vi "CameraSobelEdgeDetection.vi"() -> (4 "图像时间戳":u32=16532020 format="%_32g")   [LabVIEW 2015]
uses:
  <vilib>/Analysis/baseanly.llb/Mean (DBL).vi
  <vilib>/Instr/_visa.llb/VISA Configure Serial Port (Instr).vi
  MVCAMSDK.dll
  <vilib>/Analysis/NI_AALBase.lvlib
  <vilib>/vision/NI_Vision_Development_Module.lvlib
panel:
  out "实时循环时间":u32=16532020 format="%_32g"
  in  "平移前进 2":T1=TRUE
  in  "平移计数 2":u16
  in  "平移一次脉冲数 2":u16=20
  out "连接的字符串 2":string
  out "平移信号曲线 2":cluster{"Locations":dbl[], "Amplitudes":dbl[]}[](graph)
  out "连接的字符串":string
  out "转动信号曲线":cluster{"Locations":dbl[], "Amplitudes":dbl[]}[](graph)
  in  "平移回退":T1=TRUE
  in  "转动回退":T1=TRUE
  in  "转动计数":u16
  in  "转动一次脉冲数":u16=20
  in  "转动前进":T1=TRUE
  in  "平移一次脉冲数":u16=20
  in  "平移计数":u16
  in  "flow control (0:none)":u16(ring) caption="流控制（0:无）" items=["无", "XON/XOFF", "RTS/CTS", "XON/XOFF & RTS/CTS", "DTR/DSR", "XON/XOFF & DTR/DSR"]
  in  "stop bits (10: 1 bit)":u16=10 caption="停止位（10: 1位）"
  in  "奇偶 (0:none)":enum16{"None", "Odd", "Even", "Mark", "Space"}(ring) caption="奇偶（0:无）"
  in  "数据比特(默认8)":u16(ring)=8 items=["5"=5, "6"=6, "7"=7, "8"=8]
  in  "波特率(默认9600)":u32=9600
  in  "端口":refnum<visa-resource-name>="COM1"
  in  "平移前进":T1=TRUE
  out "泰伯距离数值":dbl[](array[numeric])=[15.393849374426454, 15.239052716055017, 15.197063981826837, 15.002070246239633]
  out "Locations":dbl[](array[numeric])=[10.438621227921368, 25.832470602347822, 41.07152331840284, 56.268587300229676, 71.27065754646931] caption="上面图像曲线波峰位置"
  out "平移信号曲线":cluster{"Locations":dbl[], "Amplitudes":dbl[]}[](graph)
  out "相机图像":T2(plugin-control)
  out "帧速":u32
  out "帧间耗时\n单位：（0.1ms）":u32
  in  "相机枚举":T3(ring)
  in  "自动曝光模式":bool=TRUE caption="软触发"
  in  "手动曝光模式":bool caption="软触发"
  in  "曝光时间，单位微秒":dbl=11000.0 format="%#_6f"
  in  "硬触发模式":bool caption="软触发"
  in  "软触发模式":bool caption="软触发"
  in  "连续模式":bool caption="软触发"
  in  "软触发一帧":bool caption="软触发"
  in  "读取自定义数据":bool
  out "从相机中读出的字符串(32字节)":string
  in  "写入自定义数据":bool
  in  "要写入相机的字符串(32字节)":string
  in  "拍照":bool
  in  "相机参数":bool=TRUE
  in  "Stop":bool
  in  "激活预览":bool=TRUE
  out "Image":T2(plugin-control)
  # "相机原生分辨率设置"
  # "写入自定义数据"
  # "触发设置"
  # "曝光设置"
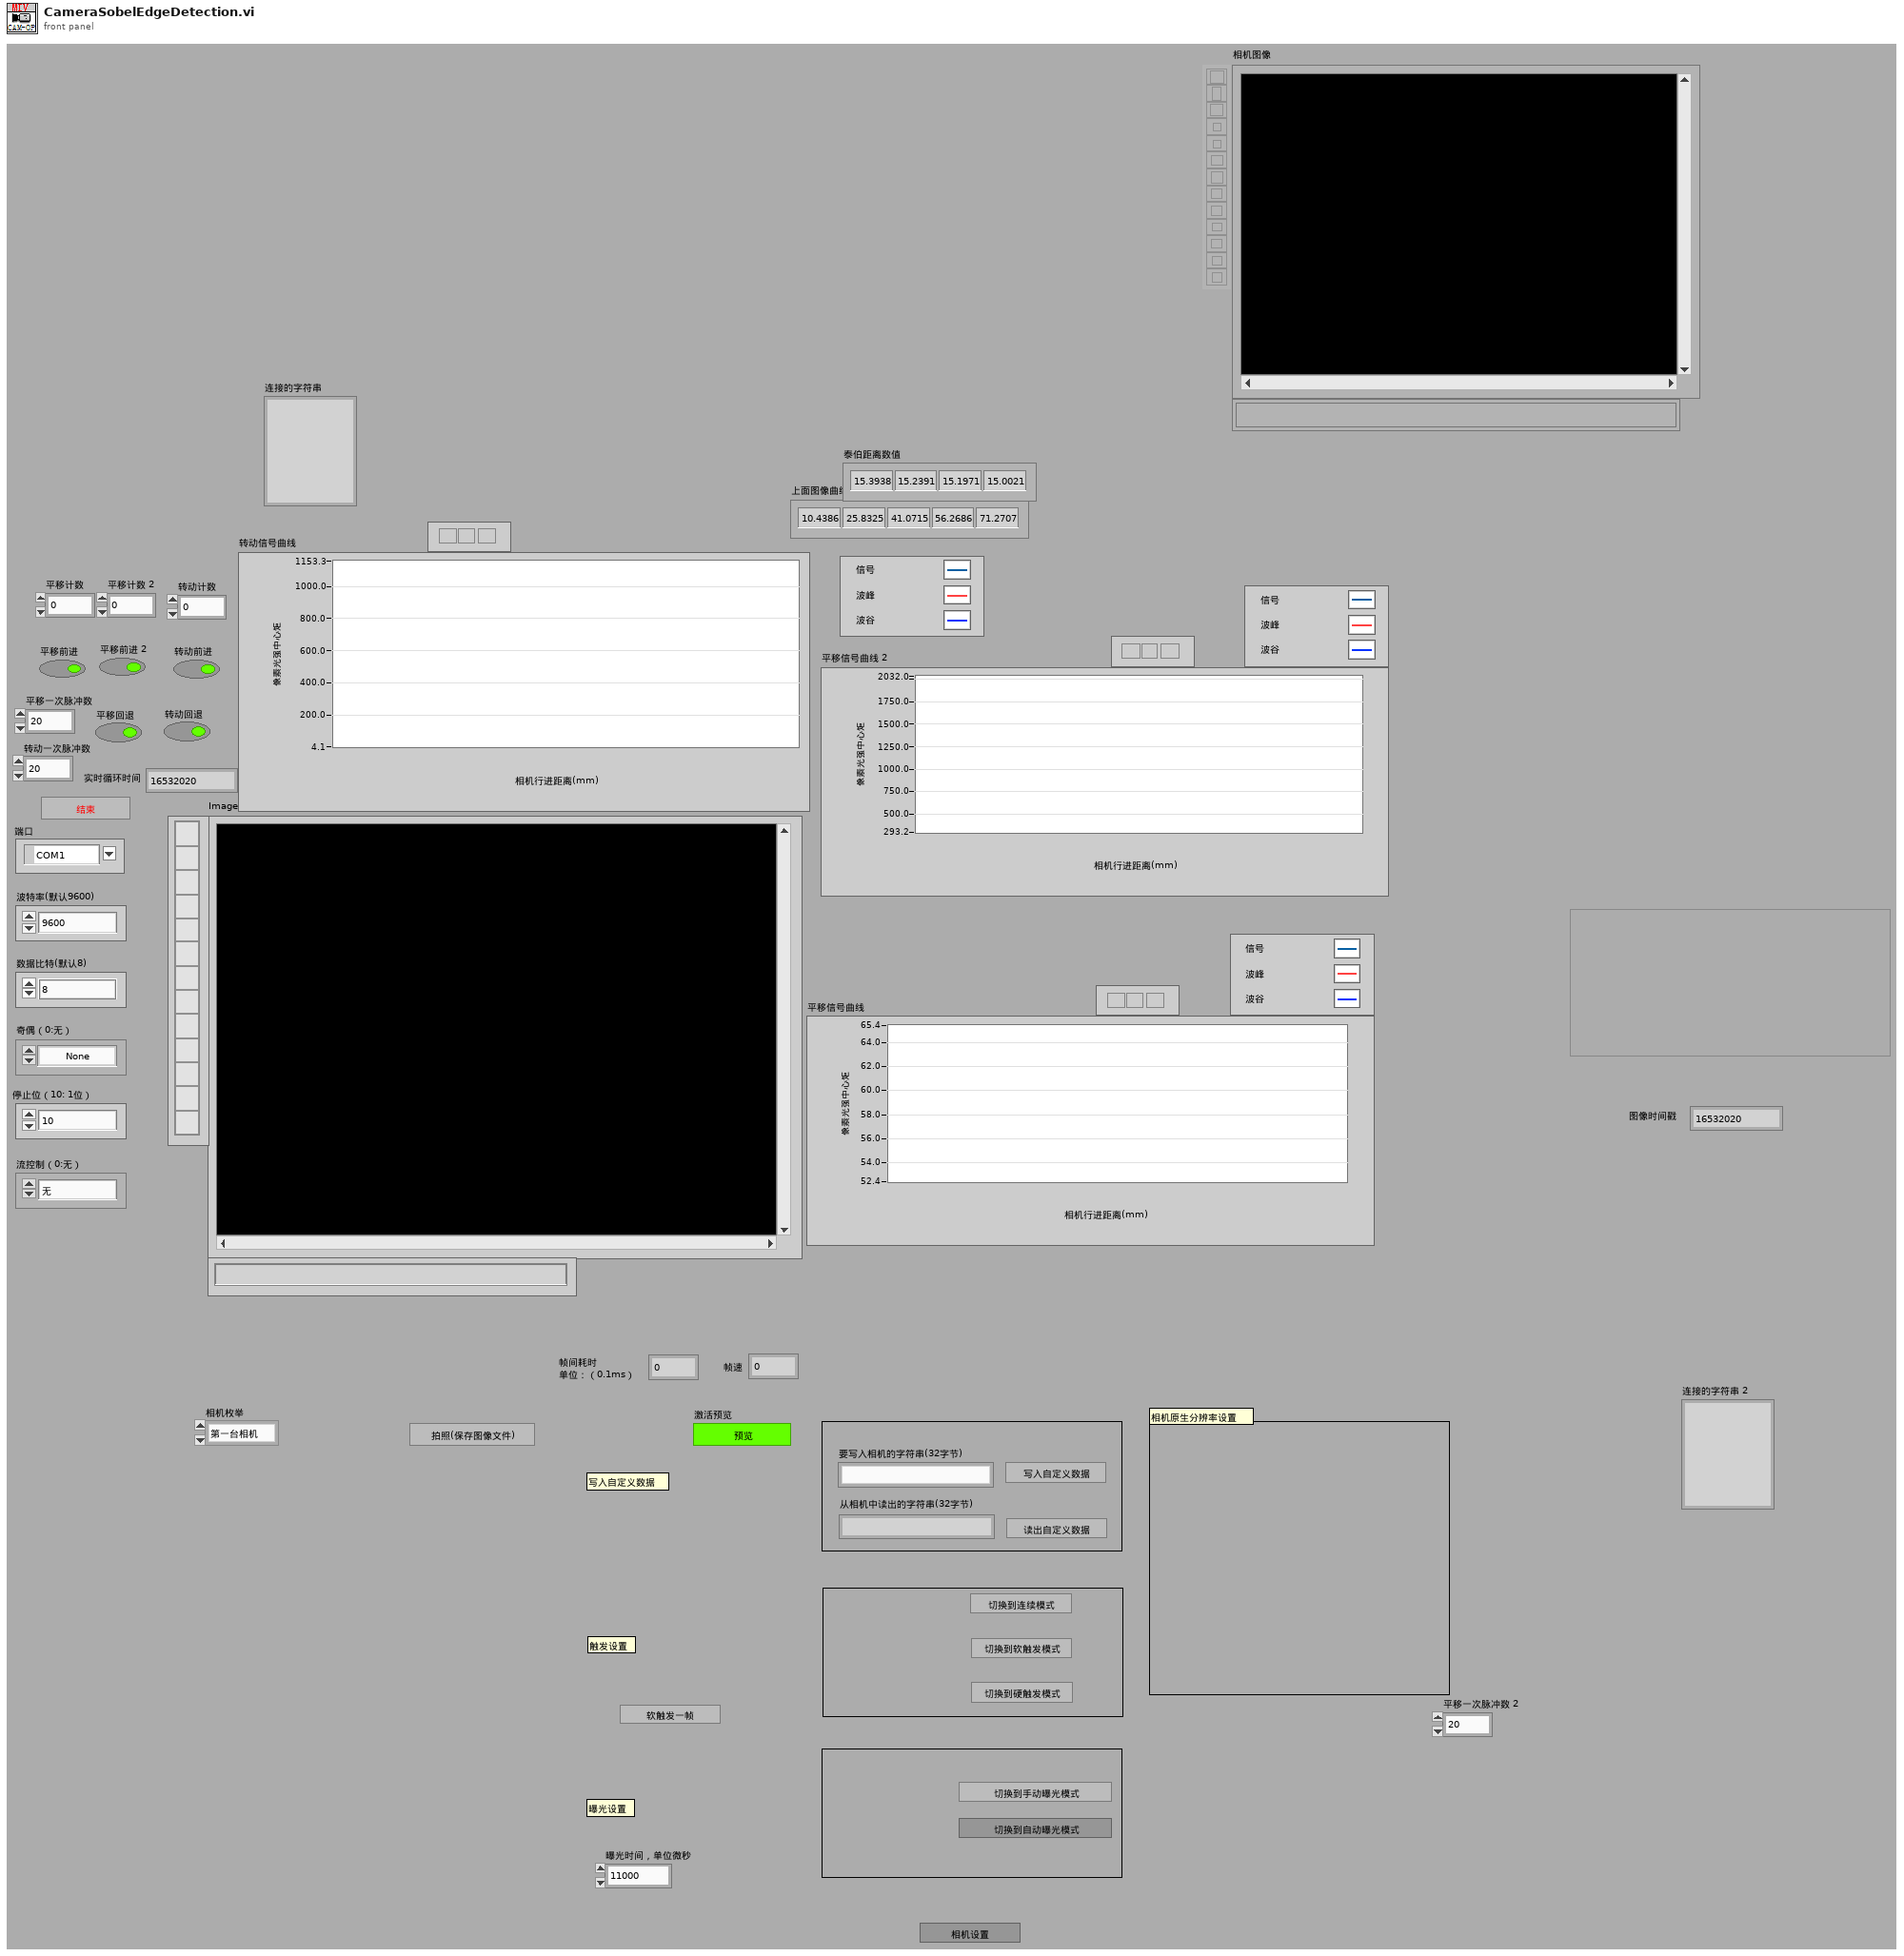
[diagram p1: front panel]
types:
  T1 = typedef "控件 1.ctl" = bool
  T2 = typedef "IMAQ Image.ctl" = refnum<image>
  T3 = enum16{"第一台相机", "第二台相机", "第三台相机", "第四台相机", "第五台相机"}
  T4 = typedef "Image Type" = u32
  T5 = enum32{"Differentiation", "Gradient", "Prewitt", "Roberts", "Sigma", "Sobel"}
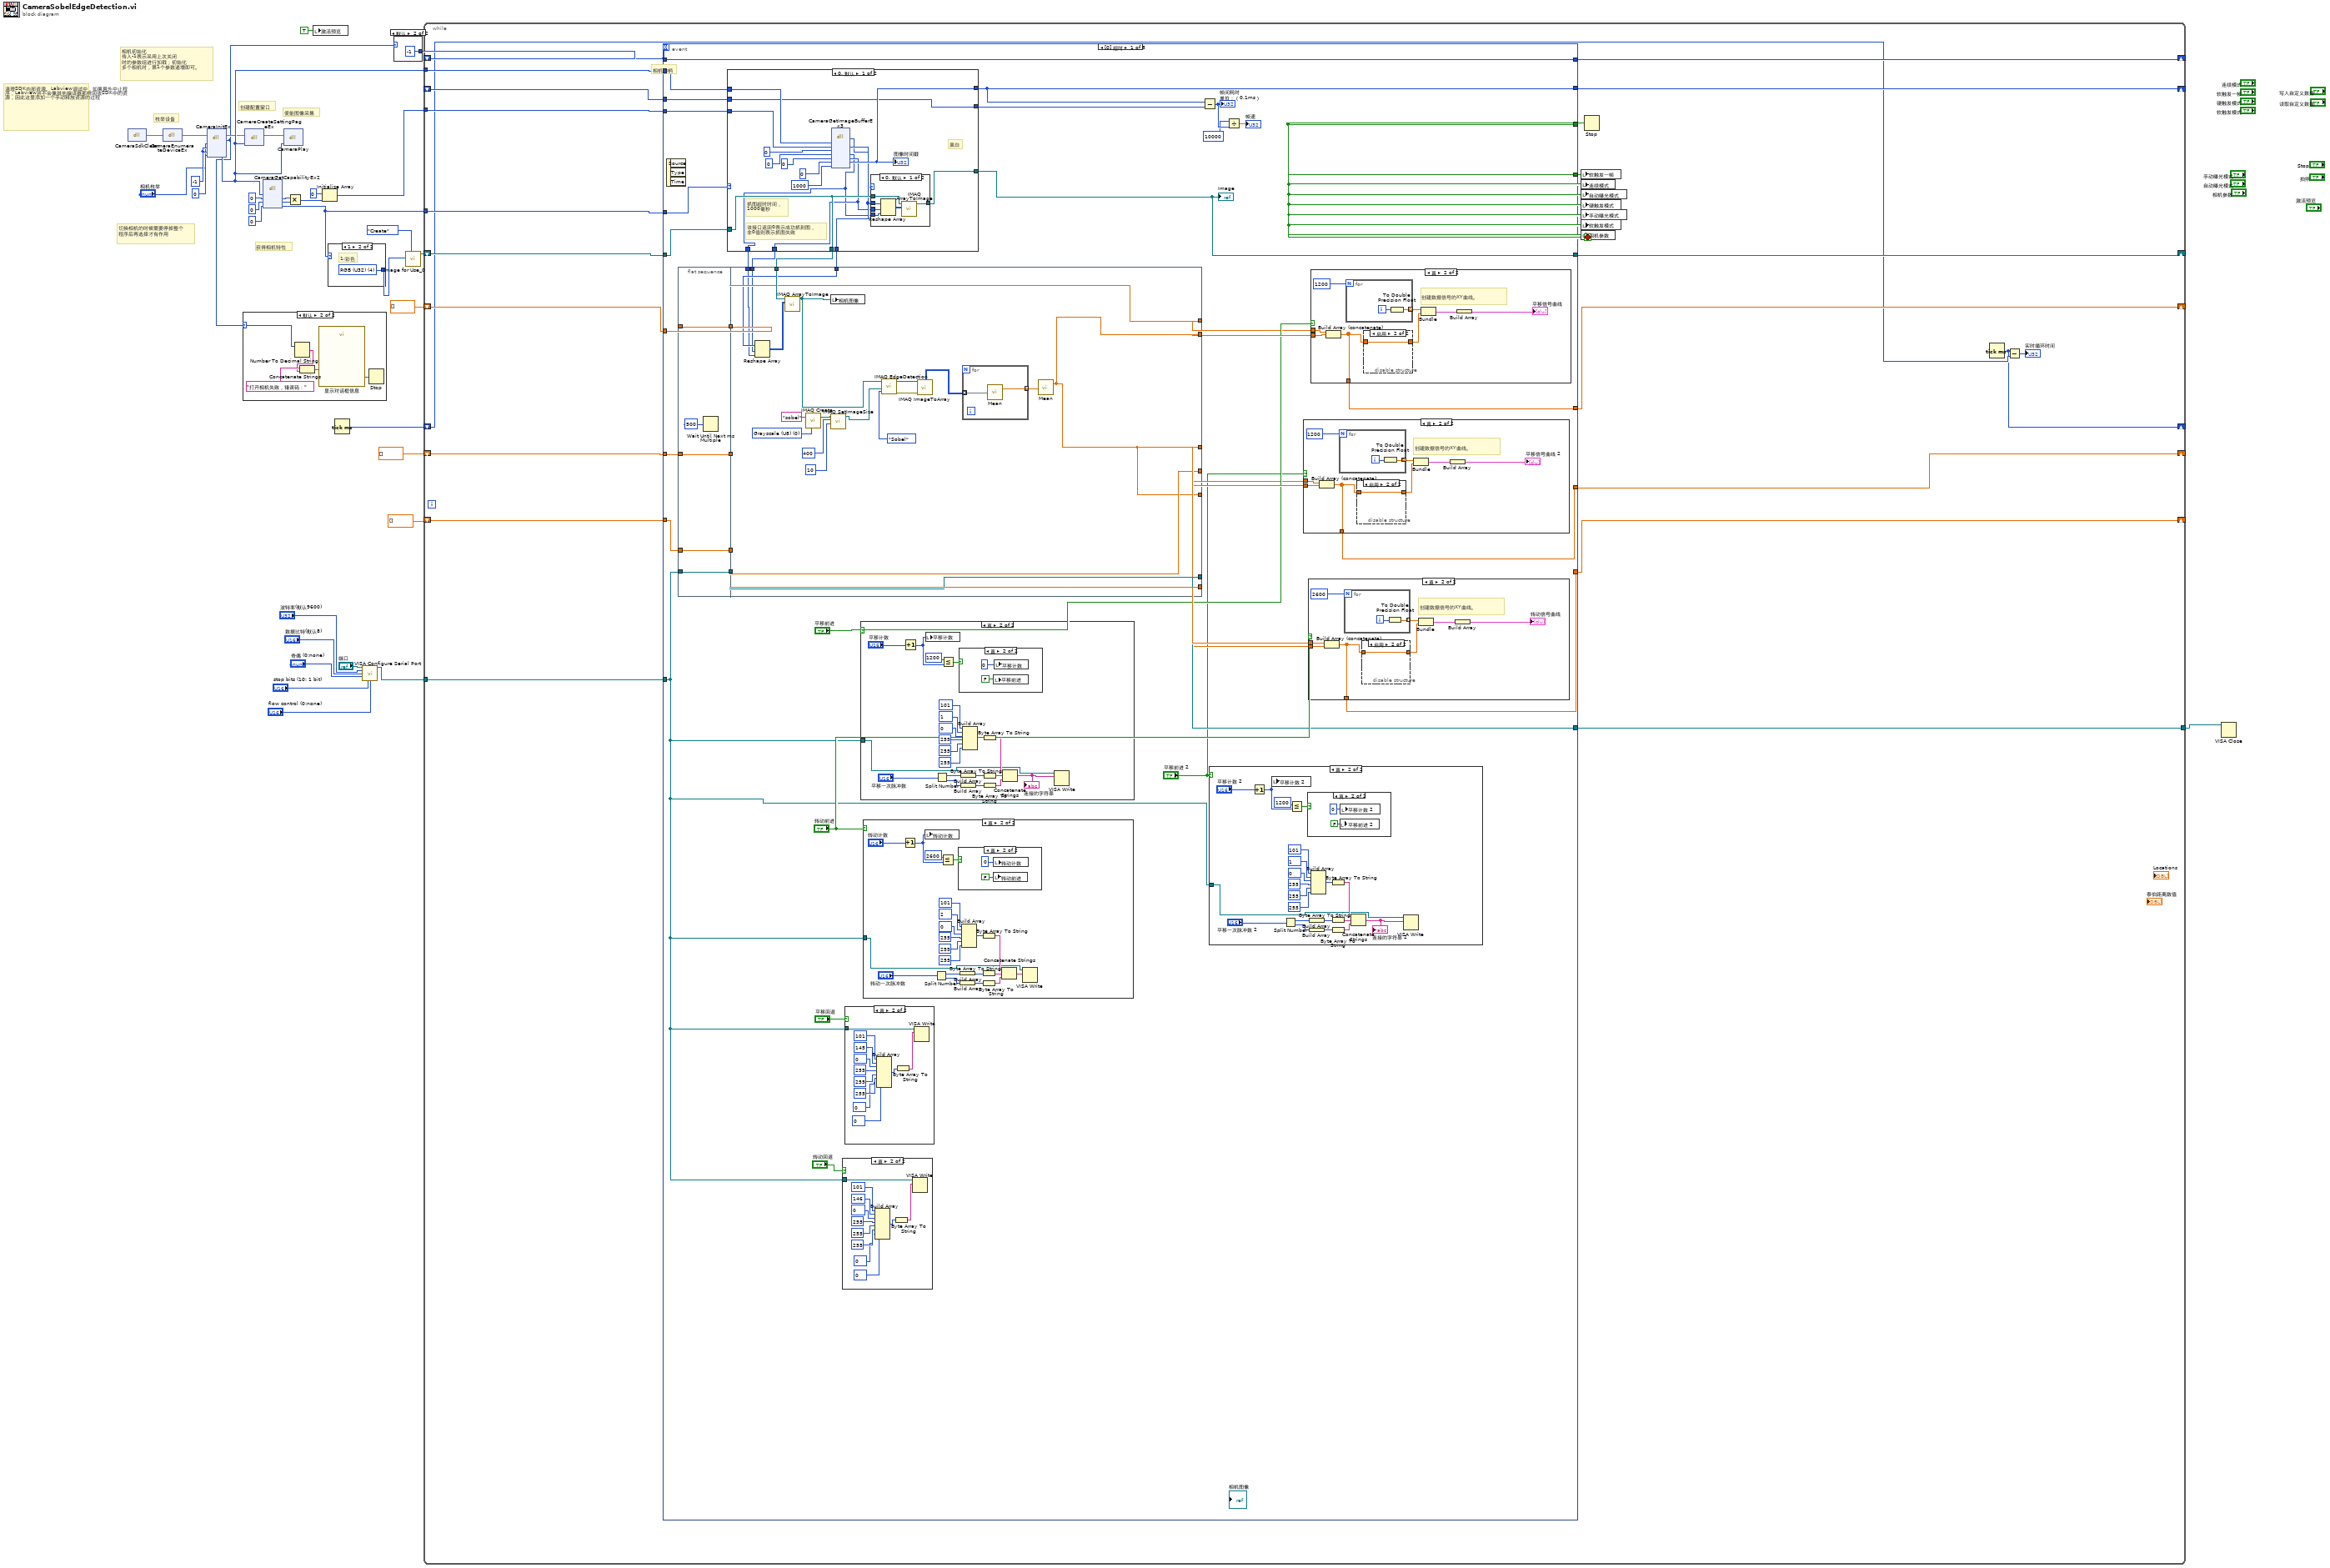
[diagram p0: block diagram]
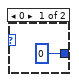
[diagram p2: hidden frame]
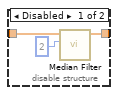
[diagram p7: hidden frame]
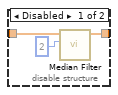
[diagram p9: hidden frame]
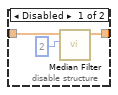
[diagram p11: hidden frame]
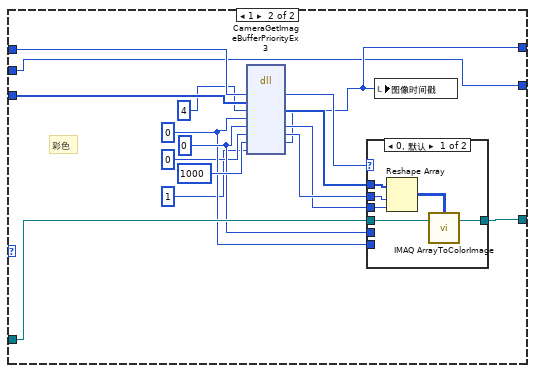
[diagram p19: hidden frame]
diagram:
  w32 = -1
  # "切换相机的时候需要停掉整个\n程序后再选择才有作用"
  # "清理SDK内部资源。Labview调试中，如果意外中止程序，Labview并不会像其他编译器那样回收SDK中的资源，因此这里添加一个手动释放资源的过程"
  # "使能图像采集"
  # "获得相机特性"
  # "创建配置窗口"
  # "相机初始化\n传入-1表示采用上次关闭\n时的参数组进行加载；初始化\n多个相机时，第1个参数递增即可。"
  # "枚举设备"
  n1 = dll-call lib="MVCAMSDK.dll" fn="CameraSdkClean"() -> (error out=w33:errorcluster)  [unwired: 4 in, 1 out]
  n2 = dll-call lib="MVCAMSDK.dll" fn="CameraEnumerateDeviceEx"(error in=w33) -> (error out=w30:errorcluster)  [unwired: 3 in, 1 out]
  n3 = dll-call lib="MVCAMSDK.dll" fn="CameraInitEx"(error in=w30, "相机索引值"="相机枚举", "参数加载方式"=w32, "要加载的参数组索引"=w32, "相机句柄"=0) -> (error out=w19:errorcluster, "返回类型"=w14:i32, "相机句柄"=w21:i32)  [unwired: 5 in, 1 out]
  n4 = case shown="默认" w14 {
    selector: w14 -> [_ w39]
    frame 0 {
    }
    frame Default {
      n5 = Number To Decimal String(number=w39) -> (decimal integer string=w36:string)  [unwired: 1 in]
      n6 = Concatenate Strings("打开相机失败，错误码：" ("字符串"), w36) -> (w38:string)
      n7 = call "显示对话框信息"("Message"=w38) -> ("结束"=w40:bool)  [unwired: 9 in, 1 out]
      n8 = Stop(stop? (T)=w40) -> ()
    }
  }
  n9 = dll-call lib="MVCAMSDK.dll" fn="CameraCreateSettingPageEx"(error in=w19, "相机句柄"=w21) -> (error out=w22:errorcluster)  [unwired: 4 in, 1 out]
  n10 = dll-call lib="MVCAMSDK.dll" fn="CameraGetCapabilityEx2"("相机句柄"=w21, "图像最大宽度"=0, "图像最大高度"=0, "是否是彩色相机(返回0:黑白;1:彩色)"=0) -> ("图像最大宽度"=w24:i32, "图像最大高度"=w23:i32, "是否是彩色相机(返回0:黑白;1:彩色)"=w18:i32)  [unwired: 5 in, 2 out]
  n11 = dll-call lib="MVCAMSDK.dll" fn="CameraPlay"(error in=w22, "相机句柄"=w21) -> ()  [unwired: 4 in, 2 out]
  n12 = Multiply(x=w24, y=w23) -> (x*y=w28:i32)
  n13 = local write "激活预览"(TRUE ("激活预览")) -> ()
  n14 = Initialize Array(0, w28) -> (w20:i32[])
  n15 = case shown="1" w18 {
    tunnel: [_ w41] -> w34
    frame 0, Default {
      # "0:黑白;"
    }
    frame 1 {
      w41 = T4 4 items=["Grayscale (U8)", "Grayscale (I16)", "Grayscale (SGL)", "Complex (CSG)", "RGB (U32)", "HSL (U32)", "RGB (U64)", "Grayscale (U16)"] ("Image Type")
      # "1:彩色"
    }
  }
  n16 = Tick Count (ms)() -> (millisecond timer value=w1:u32)
  n17 = call-poly "VISA Configure Serial Port"("VISA resource name"="端口", "baud rate (9600)"="波特率(默认9600)", "data bits (8)"="数据比特(默认8)", "parity (0:none)"="奇偶 (0:none)", "stop bits (10: 1 bit)"="stop bits (10: 1 bit)", "flow control (0:none)"="flow control (0:none)") -> ("VISA resource name out"=w6:refnum<visa-resource-name>)  [unwired: 8 in, 1 out]
  n18 = case shown="默认" w14 {
    tunnel: [0 -1] -> w13
    frame 0 {
    }
    frame Default {
    }
  }
  n19 = call "Image for Use_0.vi"("Command"=enum16{"Create", "Use", "Copy in", "Dispose"}."Create", "Image Type"=w34) -> ("Image out"=w17:T2)  [unwired: 8 in, 1 out]
  n20 = while {
    tunnel: w21 -> [w62]
    tunnel: w20 -> [w64]
    tunnel: w18 -> [w65]
    shift-right: [w61] -> _
    shift-left: w13 -> [w60]
    shift-right: [w58] -> _
    shift-left: w17 -> [w63]
    shift-right: [w57] -> _
    shift-left: _ -> [w56]
    tunnel: w6 -> [w54]
    tunnel: [w53] -> w5
    shift-right: [w51] -> _
    shift-left: dbl[] [] -> [w52]
    shift-right: [w50] -> _
    shift-left: dbl[] [] -> [w49]
    shift-right: [w47] -> _
    shift-left: dbl[] [] -> [w48]
    shift-right: [w44] -> _
    shift-left: w1 -> [w45]
    stop <- w55 stop-if-true
    # "相机句柄"
    n21 = event shown="[0] 超时" {
      selector: _ -> [_ _ _ _ _ _ _ _]
      dyn-events: _ -> [_ _ _ _ _ _ _ _]
      timeout: w60 -> [_ _ _ _ _ _ _ _]
      tunnel: [_ _ _ _ _ _ _ TRUE] -> w55
      tunnel: w64 -> [w103 _ _ _ _ _ _ _]
      tunnel: w65 -> [w102 _ _ _ _ _ _ _]
      tunnel: w62 -> [w104 _ w323 w341 w356 _ w370 w390]
      tunnel: w63 -> [w101 w316 w322 w340 w355 w360 w369 w388]
      tunnel: [w100 w317 w324 w342 w357 w361 w371 w391] -> w61
      tunnel: w60 -> [w100 _ w324 w342 w357 w361 w371 w391]
      tunnel: [_ _ _ _ _ _ _ FALSE] -> w59
      tunnel: [w99 w316 w322 w340 w355 w360 w369 w388] -> w58
      tunnel: [w96 w315 w321 w339 w354 w359 w368 w387] -> w57
      tunnel: w56 -> [w98 w315 w321 w339 w354 w359 w368 w387]
      tunnel: w54 -> [w69 _ _ _ _ _ _ _]
      tunnel: [w80 _ _ _ _ _ _ _] -> w53
      tunnel: w52 -> [w86 _ _ _ _ _ _ _]
      tunnel: [w89 _ _ _ _ _ _ _] -> w51
      tunnel: [w88 _ _ _ _ _ _ _] -> w50
      tunnel: w49 -> [w82 _ _ _ _ _ _ _]
      tunnel: [w77 _ _ _ _ _ _ _] -> w47
      tunnel: w48 -> [w74 _ _ _ _ _ _ _]
      event Timeout {
        n22 = event-data() -> ()  [unwired: 1 in, 3 out]
        n23 = flat-sequence {
          tunnel: w86 -> [w147]
          tunnel: [w147] -> w85
          tunnel: [w145] -> w83
          tunnel: w82 -> [w145]
          tunnel: [w144] -> w81
          tunnel: w69 -> [w144]
          tunnel: w74 -> [w143]
          tunnel: [w143] -> w73
          tunnel: w92 -> [w169]
          tunnel: [w157] -> w78
          tunnel: [w168] -> w71
          tunnel: w85 -> [w168]
          tunnel: [w167] -> w84
          tunnel: w83 -> [w167]
          tunnel: [w166] -> w80
          tunnel: w81 -> [w166]
          tunnel: [w157] -> w79
          tunnel: [w157] -> w76
          tunnel: w73 -> [w165]
          tunnel: [w165] -> w72
          tunnel: w68 -> [w150]
          tunnel: w67 -> [w149]
          tunnel: w66 -> [w148]
          frame #0 {
            n24 = Wait Until Next ms Multiple(millisecond multiple=u32 500 ("毫秒倍数")) -> ()  [unwired: 1 out]
          }
          frame #1 {
            w156 = T4 0 items=["Grayscale (U8)", "Grayscale (I16)", "Grayscale (SGL)", "Complex (CSG)", "RGB (U32)", "HSL (U32)", "RGB (U64)", "Grayscale (U16)"] ("Image Type")
            n25 = Reshape Array(w150, w149, w148) -> (w151:u8[][])
            n26 = call "IMAQ ArrayToImage"("Image Pixels (U8)"=w151, "Image"=w169) -> ("Image Out"=w160:T2)  [unwired: 8 in, 1 out]
            n27 = call "IMAQ Create"("Image Name"="sobel", "Image Type"=w156) -> ("New Image"=w155:T2)  [unwired: 3 in, 1 out]
            n28 = local write "相机图像"(w160) -> ()
            n29 = call "IMAQ SetImageSize"("Y Resolution"=10, "X Resolution"=400, "Image"=w155) -> ("Image Out"=w154:T2)  [unwired: 2 in, 1 out]
            n30 = call "IMAQ EdgeDetection"("Method"=T5."Sobel", "Image Dst"=w154, "Image Src"=w160) -> ("error out"=w161:errorcluster, "Image Dst Out"=w162:T2)  [unwired: 7 in]
            n31 = call "IMAQ ImageToArray"("error in (no error)"=w161, "Image"=w162) -> ("Image Pixels (U8)"=w159:u8[][])  [unwired: 2 in, 4 out]
            n32 = for {
              tunnel: w159 -> [w171] mode=indexing
              tunnel: [w170] -> w158 mode=indexing
              n33 = call-poly <vilib>:"Mean.vi"("X"=w171) -> ("mean"=w170:dbl)  [unwired: 1 out]
            }
            n34 = call-poly <vilib>:"Mean.vi"("X"=w158) -> ("mean"=w157:dbl)  [unwired: 1 out]
          }
        }
        n35 = case shown="0, 默认" w102 {
          tunnel: w103 -> [w284 w307]
          tunnel: w101 -> [w274 w306]
          tunnel: w104 -> [w277 w305]
          tunnel: [w278 w295] -> w99
          tunnel: [w276 w294] -> w96
          tunnel: w98 -> [w275 w293]
          tunnel: [w275 w293] -> w97
          tunnel: [w274 _] -> w92
          tunnel: [w273 _] -> w68
          tunnel: [w271 _] -> w67
          tunnel: [w270 _] -> w66
          frame 0, Default {
            # "黑白"
            # "该接口返回0表示成功抓到图，\n非0值则表示抓图失败"
            # "抓图超时时间，\n1000毫秒"
            n36 = dll-call lib="MVCAMSDK.dll" fn="CameraGetImageBufferEx3"("相机句柄"=w277, "图像数据缓冲区"=w284, "图像输出格式(0:8位灰度;1:24位彩色;2:32位彩色，3：BGR24彩色 4：BGRA32位彩色)"=0, "图像宽度"=0, "图像高度"=0, "时间戳(单位为100微秒)"=0, "抓图超时时间(毫秒)"=1000) -> ("返回类型"=w272:i32, "图像数据缓冲区"=w273:u8[], "图像宽度"=w270:i32, "图像高度"=w271:i32, "时间戳(单位为100微秒)"=w276:u32)  [unwired: 6 in, 2 out]
            "图像时间戳" <- w276
            n37 = case shown="0, 默认" w272 {
              tunnel: w273 -> [w290 _]
              tunnel: w274 -> [w287 w291]
              tunnel: w271 -> [w289 _]
              tunnel: w270 -> [w288 _]
              tunnel: [w285 w291] -> w278
              frame 0, Default {
                n38 = Reshape Array(w290, w289, w288) -> (w286:u8[][])
                n39 = call "IMAQ ArrayToImage"("Image Pixels (U8)"=w286, "Image"=w287) -> ("Image Out"=w285:T2)  [unwired: 8 in, 1 out]
              }
              frame -12 {
              }
            }
          }
          frame 1 {
            w297 = 0
            w298 = 0
            # "彩色"
            n40 = dll-call lib="MVCAMSDK.dll" fn="CameraGetImageBufferPriorityEx3"("相机句柄"=w305, "图像数据缓冲区"=w307, "图像输出格式(0:8位灰度;1:24位彩色;2:32位彩色)"=4, "图像宽度"=w297, "图像高度"=w298, "时间戳（单位为100微秒）"=0, "抓图超时时间(毫秒)"=1000, "取图优先级(0: 取最旧   1:取最新)"=1) -> ("返回类型"=w299:i32, "图像数据缓冲区"=w302:u32[], "图像宽度"=w300:i32, "图像高度"=w301:i32, "时间戳（单位为100微秒）"=w294:u32)  [unwired: 7 in, 2 out]
            n41 = case shown="0, 默认" w299 {
              tunnel: w302 -> [w312 _]
              tunnel: w306 -> [w311 w314]
              tunnel: w301 -> [w310 _]
              tunnel: w300 -> [w309 _]
              tunnel: w298 -> [_ _]
              tunnel: w297 -> [_ _]
              tunnel: [w308 w314] -> w295
              frame 0, Default {
                n42 = Reshape Array(w312, w310, w309) -> (w313:u32[][])
                n43 = call "IMAQ ArrayToColorImage"("Image Pixels (U32)"=w313, "Image"=w311) -> ("Image Out"=w308:T2)  [unwired: 3 in, 1 out]
              }
              frame -12 {
              }
            }
            n44 = local write "图像时间戳"(w294) -> ()
          }
        }
        "Image" <- w99
        n45 = case shown="真" "转动回退" {
          tunnel: w69 -> [_ w205]
          frame False {
          }
          frame True {
            n46 = Build Array(101, 146, 0, 255, 255, 255, 0, 0) -> (w206:i32[])
            n47 = Byte Array To String(unsigned byte array=w206) -> (string=w204:string)
            n48 = VISA Write(VISA resource name=w205, write buffer=w204) -> ()  [unwired: 1 in, 3 out]
          }
        }
        n49 = case shown="真" "平移回退" {
          tunnel: w69 -> [_ w216]
          frame False {
          }
          frame True {
            n50 = Build Array(101, 145, 0, 255, 255, 255, 0, 0) -> (w217:i32[])
            n51 = Byte Array To String(unsigned byte array=w217) -> (string=w215:string)
            n52 = VISA Write(VISA resource name=w216, write buffer=w215) -> ()  [unwired: 1 in, 3 out]
          }
        }
        n53 = case shown="真" "平移前进" {
          tunnel: w69 -> [_ w250]
          frame False {
          }
          frame True {
            n54 = Increment(x="平移计数") -> (x+1=w248:u16)
            n55 = local write "平移计数"(w248) -> ()
            n56 = Split Number(x="平移一次脉冲数") -> (hi(x)=w258:u8, lo(x)=w257:u8)
            n57 = Less Or Equal?(x=1200, y=w248) -> (x <= y?=w260:bool)
            n58 = case shown="真" w260 {
              frame False {
              }
              frame True {
                n59 = local write "平移前进"(T1 FALSE ("平移前进")) -> ()
                n60 = local write "平移计数"(u16 0 ("平移计数 2")) -> ()
              }
            }
            n61 = Build Array(w258) -> (w256:u8[])
            n62 = Build Array(w257) -> (w255:u8[])
            n63 = Build Array(101, 1, 0, 255, 255, 255) -> (w254:i32[])
            n64 = Byte Array To String(unsigned byte array=w254) -> (string=w253:string)
            n65 = Byte Array To String(unsigned byte array=w256) -> (string=w252:string)
            n66 = Byte Array To String(unsigned byte array=w255) -> (string=w251:string)
            n67 = Concatenate Strings(w253, w252, w251) -> (w247:string)
            "连接的字符串" <- w247
            n68 = VISA Write(VISA resource name=w250, write buffer=w247) -> ()  [unwired: 1 in, 3 out]
          }
        }
        n69 = case shown="真" "转动前进" {
          tunnel: w69 -> [_ w228]
          frame False {
          }
          frame True {
            n70 = Increment(x="转动计数") -> (x+1=w226:u16)
            n71 = local write "转动计数"(w226) -> ()
            n72 = Split Number(x="转动一次脉冲数") -> (hi(x)=w236:u8, lo(x)=w235:u8)
            n73 = Less Or Equal?(x=2600, y=w226) -> (x <= y?=w238:bool)
            n74 = case shown="真" w238 {
              frame False {
              }
              frame True {
                n75 = local write "转动前进"(T1 FALSE ("平移前进")) -> ()
                n76 = local write "转动计数"(u16 0 ("平移计数")) -> ()
              }
            }
            n77 = Build Array(w236) -> (w234:u8[])
            n78 = Build Array(w235) -> (w233:u8[])
            n79 = Build Array(101, 2, 0, 255, 255, 255) -> (w232:i32[])
            n80 = Byte Array To String(unsigned byte array=w232) -> (string=w231:string)
            n81 = Byte Array To String(unsigned byte array=w234) -> (string=w230:string)
            n82 = Byte Array To String(unsigned byte array=w233) -> (string=w229:string)
            n83 = Concatenate Strings(w231, w230, w229) -> (w225:string)
            n84 = VISA Write(VISA resource name=w228, write buffer=w225) -> ()  [unwired: 1 in, 3 out]
          }
        }
        n85 = Subtract(x=w96, y=w97) -> (x-y=w95:u32)
        "帧间耗时\n单位：（0.1ms）" <- w95
        n86 = case shown="真" "平移前进 2" {
          tunnel: w69 -> [_ w108]
          frame False {
          }
          frame True {
            n87 = Increment(x="平移计数 2") -> (x+1=w106:u16)
            n88 = local write "平移计数 2"(w106) -> ()
            n89 = Split Number(x="平移一次脉冲数 2") -> (hi(x)=w116:u8, lo(x)=w115:u8)
            n90 = Less Or Equal?(x=1200, y=w106) -> (x <= y?=w118:bool)
            n91 = case shown="真" w118 {
              frame False {
              }
              frame True {
                n92 = local write "平移前进 2"(T1 FALSE ("平移前进")) -> ()
                n93 = local write "平移计数 2"(u16 0 ("平移计数 2")) -> ()
              }
            }
            n94 = Build Array(w116) -> (w114:u8[])
            n95 = Build Array(w115) -> (w113:u8[])
            n96 = Build Array(101, 1, 0, 255, 255, 255) -> (w112:i32[])
            n97 = Byte Array To String(unsigned byte array=w112) -> (string=w111:string)
            n98 = Byte Array To String(unsigned byte array=w114) -> (string=w110:string)
            n99 = Byte Array To String(unsigned byte array=w113) -> (string=w109:string)
            n100 = Concatenate Strings(w111, w110, w109) -> (w105:string)
            "连接的字符串 2" <- w105
            n101 = VISA Write(VISA resource name=w108, write buffer=w105) -> ()  [unwired: 1 in, 3 out]
          }
        }
        n102 = Divide(x=u32 10000 ("帧间耗时"), y=w95) -> (x/y=→"帧速":dbl)
        n103 = case shown="真" "平移前进 2" {
          tunnel: w72 -> [w128 w131]
          tunnel: w76 -> [_ w129]
          tunnel: [w128 w130] -> w77
          frame False {
          }
          frame True {
            # "创建数据信号的XY曲线。"
            n104 = Build Array (concatenate)(w131, w129) -> (w130:dbl[])
            n105 = for {
              N: i64 1200 ("数值") -> [_]
              tunnel: [w137] -> w135 mode=indexing
              i -> [w138]
              n106 = To Double Precision Float(number=w138) -> (double precision float=w137:dbl)
            }
            n107 = disable-structure shown="启用" {
              disable-tunnel: w130 -> [w140 w142]
              disable-tunnel: [w139 w142] -> w134
              frame Disabled {
                n108 = call <vilib>:"Median Filter.vi"("left rank"=2, "X"=w140) -> ("Filtered X"=w139:dbl[])  [unwired: 8 in, 1 out]
              }
              frame Enabled {
              }
            }
            n109 = Bundle(w135, w134) -> (w132:cluster{dbl[], dbl[]})  [unwired: 1 in]
            n110 = Build Array(w132) -> (→"平移信号曲线 2":cluster{dbl[], dbl[]}[])
          }
        }
        n111 = case shown="真" "转动前进" {
          tunnel: w79 -> [_ w175]
          tunnel: w84 -> [w172 w174]
          tunnel: [w172 w173] -> w88
          frame False {
          }
          frame True {
            # "创建数据信号的XY曲线。"
            n112 = Build Array (concatenate)(w174, w175) -> (w173:dbl[])
            n113 = for {
              N: i64 2600 ("数值") -> [_]
              tunnel: [w181] -> w177 mode=indexing
              i -> [w182]
              n114 = To Double Precision Float(number=w182) -> (double precision float=w181:dbl)
            }
            n115 = disable-structure shown="启用" {
              disable-tunnel: w173 -> [w184 w186]
              disable-tunnel: [w183 w186] -> w178
              frame Disabled {
                n116 = call <vilib>:"Median Filter.vi"("left rank"=2, "X"=w184) -> ("Filtered X"=w183:dbl[])  [unwired: 8 in, 1 out]
              }
              frame Enabled {
              }
            }
            n117 = Bundle(w177, w178) -> (w180:cluster{dbl[], dbl[]})  [unwired: 1 in]
            n118 = Build Array(w180) -> (→"转动信号曲线":cluster{dbl[], dbl[]}[])
          }
        }
        n119 = case shown="真" "平移前进" {
          tunnel: w71 -> [w187 w189]
          tunnel: w78 -> [_ w190]
          tunnel: [w187 w188] -> w89
          frame False {
          }
          frame True {
            # "创建数据信号的XY曲线。"
            n120 = Build Array (concatenate)(w189, w190) -> (w188:dbl[])
            n121 = for {
              N: i64 1200 ("数值") -> [_]
              tunnel: [w196] -> w194 mode=indexing
              i -> [w197]
              n122 = To Double Precision Float(number=w197) -> (double precision float=w196:dbl)
            }
            n123 = disable-structure shown="启用" {
              disable-tunnel: w188 -> [w199 w201]
              disable-tunnel: [w198 w201] -> w193
              frame Disabled {
                n124 = call <vilib>:"Median Filter.vi"("left rank"=2, "X"=w199) -> ("Filtered X"=w198:dbl[])  [unwired: 8 in, 1 out]
              }
              frame Enabled {
              }
            }
            n125 = Bundle(w194, w193) -> (w191:cluster{dbl[], dbl[]})  [unwired: 1 in]
            n126 = Build Array(w191) -> (→"平移信号曲线":cluster{dbl[], dbl[]}[])
          }
        }
      }
      event "激活预览": Value Change {
        n127 = event-data() -> ("NewVal"=w318:bool)  [unwired: 1 in, 5 out]
        n128 = case shown="真" w318 {
          tunnel: [-1 0] -> w317
          frame False {
          }
          frame True {
          }
        }
      }
      event "连续模式", "软触发一帧", "硬触发模式", "软触发模式": Value Change {
        n129 = event-data() -> ("CtlRef"=w326:refnum<vi>)  [unwired: 1 in, 5 out]
        n130 = control-ref of="连续模式"() -> (w328:refnum<vi>)
        n131 = control-ref of="硬触发模式"() -> (w329:refnum<vi>)
        n132 = control-ref of="软触发模式"() -> (w330:refnum<vi>)
        n133 = control-ref of="软触发一帧"() -> (w331:refnum<vi>)
        n134 = Build Array ("创建数组")(w328, w329, w330, w331) -> (w327:refnum<vi>[])
        n135 = Search 1D Array(1D array=w327, element=w326) -> (index of element=w325:i32)  [unwired: 1 in]
        n136 = case shown="1" w325 {
          tunnel: w323 -> [w332 w334 w336 w338]
          frame 0, Default {
            # "连续模式"
            n137 = dll-call lib="MVCAMSDK.dll" fn="CameraSetTriggerMode"("相机句柄"=w332, "模式"=0) -> ()  [unwired: 6 in, 2 out]
          }
          frame 1 {
            # "硬触发模式"
            n138 = dll-call lib="MVCAMSDK.dll" fn="CameraSetTriggerMode"("相机句柄"=w334, "模式"=2) -> ()  [unwired: 6 in, 2 out]
          }
          frame 2 {
            # "软触发模式"
            n139 = dll-call lib="MVCAMSDK.dll" fn="CameraSetTriggerMode"("相机句柄"=w336, "模式"=1) -> ()  [unwired: 6 in, 2 out]
          }
          frame 3 {
            # "软触发一帧"
            n140 = dll-call lib="MVCAMSDK.dll" fn="CameraSoftTrigger"("相机句柄"=w338) -> ()  [unwired: 5 in, 2 out]
          }
        }
      }
      event "手动曝光模式", "自动曝光模式": Value Change {
        n141 = event-data() -> ("CtlRef"=w345:refnum<vi>)  [unwired: 1 in, 5 out]
        n142 = control-ref of="自动曝光模式"() -> (w343:refnum<vi>)
        n143 = control-ref of="手动曝光模式"() -> (w346:refnum<vi>)
        n144 = Build Array ("创建数组")(w346, w343) -> (w347:refnum<vi>[])
        n145 = Search 1D Array(1D array=w347, element=w345) -> (index of element=w344:i32)  [unwired: 1 in]
        n146 = case shown="0, 默认" w344 {
          tunnel: w341 -> [w348 w352]
          frame 0, Default {
            # "手动曝光模式"
            n147 = dll-call lib="MVCAMSDK.dll" fn="CameraSetAeState"("相机句柄"=w348, "曝光模式(0手动，1自动)"=0) -> (error out=w351:errorcluster)  [unwired: 6 in, 1 out]
            n148 = dll-call lib="MVCAMSDK.dll" fn="CameraSetExposureTime"(error in=w351, "相机句柄"=w348, "曝光时间，单位微秒"="曝光时间，单位微秒") -> ()  [unwired: 5 in, 2 out]
          }
          frame 1 {
            # "自动曝光模式"
            n149 = dll-call lib="MVCAMSDK.dll" fn="CameraSetAeState"("相机句柄"=w352, "曝光模式(0手动，1自动)"=1) -> ()  [unwired: 6 in, 2 out]
          }
        }
      }
      event "相机参数": Value Change {
        n150 = event-data() -> ()  [unwired: 1 in, 6 out]
        n151 = dll-call lib="MVCAMSDK.dll" fn="CameraShowSettingPage"("相机句柄"=w356, "状态"=TRUE) -> ()  [unwired: 6 in, 2 out]
      }
      event "拍照": Value Change {
        n152 = event-data() -> ()  [unwired: 1 in, 6 out]
        n153 = local read "Image"() -> (w362:T2)
        n154 = Format Date/Time String(time format string (%c)="%Y-%m-%d %H：%M：%S.bmp ") -> (date/time string=w366:string)  [unwired: 2 in]
        n155 = Concatenate Strings("c:\\", w366) -> (w363:string)
        n156 = String To Path(string=w363) -> (path=w365:path)
        n157 = call-poly "IMAQ Write File 2"("File Path"=w365, "Image"=w362) -> ()  [unwired: 8 in, 2 out]
      }
      event "写入自定义数据", "读取自定义数据": Value Change {
        n158 = event-data() -> ("CtlRef"=w373:refnum<vi>)  [unwired: 1 in, 5 out]
        n159 = control-ref of="读取自定义数据"() -> (w375:refnum<vi>)
        n160 = control-ref of="写入自定义数据"() -> (w374:refnum<vi>)
        n161 = Build Array ("创建数组")(w375, w374) -> (w376:refnum<vi>[])
        n162 = Search 1D Array(1D array=w376, element=w373) -> (index of element=w372:i32)  [unwired: 1 in]
        n163 = case shown="0, 默认" w372 {
          tunnel: w370 -> [w377 w384]
          frame 0, Default {
            n164 = Initialize Array(0, 32) -> (w381:i32[])
            n165 = dll-call lib="MVCAMSDK.dll" fn="CameraReadSN"("相机句柄"=w377, "序列号"=w381, "序列号级别，[0,1,2],0级为只读，1,2级可写"=1) -> ("序列号"=w379:u8[])  [unwired: 6 in, 2 out]
            n166 = Byte Array To String(unsigned byte array=w379) -> (string=→"从相机中读出的字符串(32字节)":string)
          }
          frame 1 {
            n167 = dll-call lib="MVCAMSDK.dll" fn="CameraWriteSN"("相机句柄"=w384, "序列号(固定为32个字节)"="要写入相机的字符串(32字节)", "序列号级别，[0,1,2]对应3级序列号，其中0级为只读，1,2级可写"=1) -> ()  [unwired: 7 in, 2 out]
          }
        }
      }
      event "Stop": Value Change {
        # "反初始化相机"
        n168 = event-data() -> ()  [unwired: 1 in, 6 out]
        n169 = dll-call lib="MVCAMSDK.dll" fn="CameraUnInit"("相机句柄"=w390) -> ()  [unwired: 5 in, 2 out]
      }
    }
    n170 = local write "软触发一帧"(w59) -> ()
    n171 = local write "连续模式"(w59) -> ()
    n172 = local write "自动曝光模式"(w59) -> ()
    n173 = local write "硬触发模式"(w59) -> ()
    n174 = local write "手动曝光模式"(w59) -> ()
    n175 = local write "软触发模式"(w59) -> ()
    n176 = local write "相机参数"(w59) -> ()
    n177 = Stop(stop? (T)=w55) -> ()
    n178 = Tick Count (ms)() -> (millisecond timer value=w44:u32)
    n179 = Subtract(x=w44, y=w45) -> (x-y=→"实时循环时间":u32)
  }
  n180 = VISA Close(VISA resource name=w5) -> ()  [unwired: 1 in, 1 out]
